vi "SetNumeric.vi"(0 "reference in":refnum<class "GSharpCls.lvclass">, 1 "Numeric":dbl, 5 "error in (no error)":errorcluster) -> (14 "reference out":refnum<class "GSharpCls.lvclass">, 19 "error out":errorcluster)   [LabVIEW 2017, in "TestLibrary.lvlib" / "GSharpCls.lvclass"]
uses:
  GSharpCls.lvclass
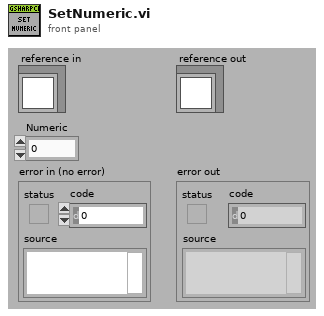
[diagram p1: front panel]
types:
  T1 = typedef "TestLibrary.lvlib/GSharpCls.lvclass/ObjectAttributesRef.ctl" = refnum<data-value>
  T2 = typedef "TestLibrary.lvlib/GSharpCls.lvclass/ObjectAttributes.ctl" = cluster{"Numeric":dbl}
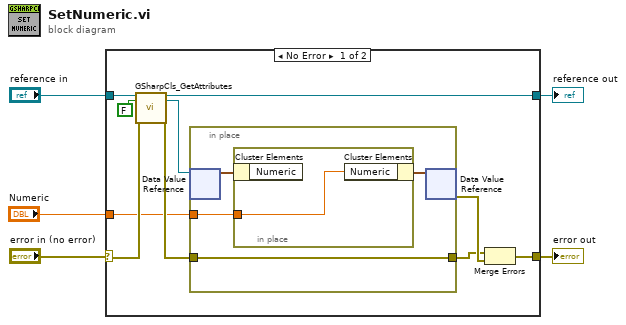
[diagram p0: block diagram]
diagram:
  n1 = case shown="No Error" "error in (no error)" {
    selector: "error in (no error)" -> [w10 w22]
    tunnel: [w15 w22] -> w4
    tunnel: [w8 w21] -> w2
    tunnel: "reference in" -> [w12 w21]
    tunnel: "Numeric" -> [w6 _]
    frame No Error {
      n2 = call "GSharpCls_GetAttributes.vi"("reference in"=w12, "return data? (T)"=FALSE, "error in (no error)"=w10) -> ("reference out"=w8:refnum<class "GSharpCls.lvclass">, "attributes ref"=w7:T1, "error out"=w9:errorcluster)  [unwired: 13 in, 1 out]
      n3 = in-place {
        in-place-border: w9 -> [w17]
        in-place-border: [w17] -> w13
        in-place-border: w6 -> [w16]
        n4 = in-place-dvr #1(w7) -> (w18:T2)  [unwired: 1 out]
        n5 = in-place {
          in-place-border: w16 -> [w20]
          n6 = in-place-cluster #2(w18) -> ()  [unwired: 1 out]
          n7 = in-place-cluster #2("Numeric"=w20) -> (w19:T2)
        }
        n8 = in-place-dvr #1(w19) -> (w14:errorcluster)  [unwired: 1 out]
      }
      n9 = Merge Errors(w13, w14) -> (w15:errorcluster)
    }
    frame Error {
    }
  }
  "error out" <- w4
  "reference out" <- w2
